vi "Merge Error.vi"(10 "Error":errorcluster, 11 "Set Error in":refnum<class "Hello World Queue.lvclass">) -> (3 "Set Error out":refnum<class "Hello World Queue.lvclass">)   [LabVIEW 2021, in "Hello World Queue.lvlib" / "Hello World Queue.lvclass"]
uses:
  Hello World Queue.lvclass
  Hello World Queue.lvclass/Hello World Queue.ctl
  Actor/Queue Actor/Queue Actor.lvclass
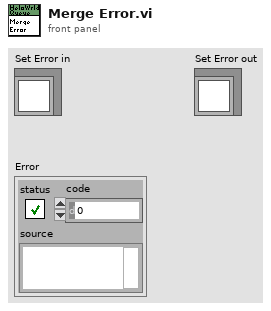
[diagram p1: front panel]
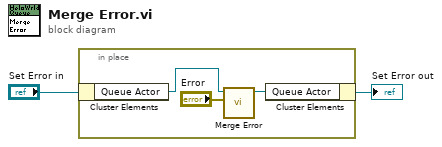
[diagram p0: block diagram]
diagram:
  n1 = in-place {
    n2 = in-place-cluster #1("Set Error in") -> ("Queue Actor"=w5:refnum<class "Queue Actor.lvclass">)
    n3 = call-dynamic "Merge Error.vi"("Error"="Error", "Set Error in"=w5) -> ("Set Error out"=w4:refnum<class "Queue Actor.lvclass">)  [unwired: 9 in]
    n4 = in-place-cluster #1("Queue Actor"=w4) -> (→"Set Error out":refnum<class "Hello World Queue.lvclass">)
  }
